vi "publish -- set -- 6.vi"(8 "request event":refnum<user-event>, 9 "response":refnum<user-event>, 10 "data":cluster{"a":dbl, "b":dbl, "c":cdb}) -> ()   [LabVIEW 2018]
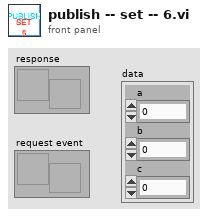
[diagram p1: front panel]
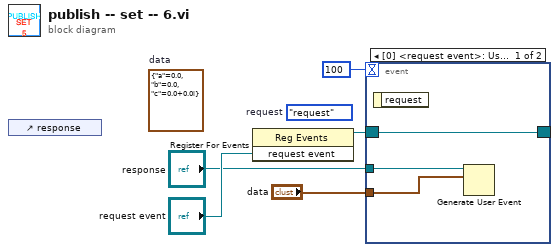
[diagram p0: block diagram]
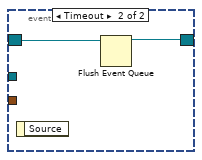
[diagram p2: hidden frame]
diagram:
  (unwired) cluster{"a":dbl, "b":dbl, "c":cdb} {"a"=0.0, "b"=0.0, "c"=0.0+0.0i}  # data
  (unwired) enum16{"request"}."request"  # request
  n1 = control-ref of="response"() -> ()  [unwired: 1 out]
  n2 = register-events("request event") -> (reference out=w5:refnum<event-registration>)  [unwired: 2 in, 1 out]
  n3 = event shown="[0] <request event>: User Event" {
    selector: w5 -> [w8 w10]
    dyn-events: [w8 w9] -> _
    timeout: 100 -> [_ _]
    tunnel: "response" -> [w7 _]
    tunnel: "data" -> [w6 _]
    event User Event {
      n4 = event-data() -> ()  [unwired: 1 in, 1 out]
      n5 = Generate User Event(user event=w7, event data cluster=w6) -> ()  [unwired: 2 in, 2 out]
    }
    event Timeout {
      n6 = event-data() -> ()  [unwired: 1 in, 1 out]
      n7 = Flush Event Queue(0:w10) -> (8:w9:refnum<event-registration>)  [unwired: 5 in, 2 out]
    }
  }
